vi "Help_w_Reg.vi"(1 "Reg No":u16, 2 "App Path":path) -> ()   [LabVIEW 2011]
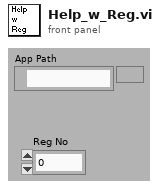
[diagram p1: front panel]
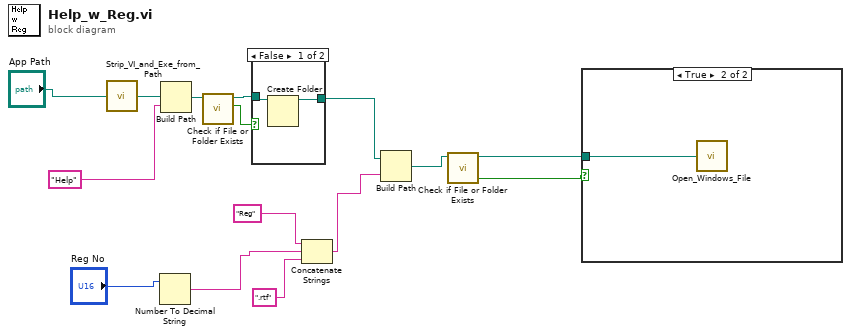
[diagram p0: block diagram]
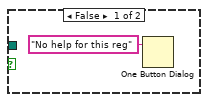
[diagram p2: hidden frame]
diagram:
  n1 = call "Strip_VI_and_Exe_from_Path.vi"("App Path"="App Path") -> ("App Path out"=w6:path)
  n2 = Number To Decimal String(number="Reg No") -> (decimal integer string=w2:string)  [unwired: 1 in]
  n3 = Build Path(base path=w6, name or relative path="Help" ("path name")) -> (appended path=w7:path)
  n4 = call <vilib>:"Check if File or Folder Exists.vi"("path"=w7) -> ("file or folder exists?"=w8:bool, "dup path"=w9:path)  [unwired: 8 in, 1 out]
  n5 = case shown="False" w8 {
    tunnel: w9 -> [w17 w18]
    tunnel: [w16 w18] -> w11
    frame False {
      n6 = Create Folder(path (use dialog)=w17) -> (created path=w16:path)  [unwired: 2 in, 2 out]
    }
    frame True {
    }
  }
  n7 = Concatenate Strings("Reg" ("name or relative path"), w2, ".rtf" ("name or relative path")) -> (w15:string)
  n8 = Build Path(base path=w11, name or relative path=w15) -> (appended path=w12:path)
  n9 = call <vilib>:"Check if File or Folder Exists.vi"("path"=w12) -> ("file or folder exists?"=w4:bool, "dup path"=w5:path)  [unwired: 8 in, 1 out]
  n10 = case shown="True" w4 {
    tunnel: w5 -> [_ w20]
    frame False {
      n11 = One Button Dialog(message="No help for this reg") -> ()  [unwired: 1 in, 1 out]
    }
    frame True {
      n12 = call "Open_Windows_File.vi"("selected path"=w20) -> ()
    }
  }
